vi "get_mcs_data.vi"(10 "MCS Parameters":T1={"Scan Length (Bins)"=64.0, "Dwell Time (s)"=1e-07, "Gate Channel Settings"={"Threshold (V)"=0.0, "Edge"=enum."Falling", "Input Impedence"=enum."1k Ohm"}, "Trig Channel Settings"={"Threshold (V)"=0.0, "Edge"=enum."Falling", "Input Impedence"=enum."1k Ohm"}, "Input 1 Settings"={"Threshold (V)"=0.0, "Edge"=enum."Falling", "Input Impedence"=enum."1k Ohm"}, "Input 2 Settings"={"Threshold (V)"=0.0, "Edge"=enum."Falling", "Input Impedence"=enum."1k Ohm"}, "Number of Sweeps"=0, "Number of Sequential Cycles"=0.0, "Number of Sequences"=0.0, "Sweep Preset"=FALSE, "Sequential Mode"=FALSE, "DAC 1 Ramp Settings"={"Ramp Mode"=enum."Fixed", "Ramp Start Value (V)"=0.0, "Ramp Length (Steps)"=1, "Step Width (bins)"=0, "Step Size (V)"=0.0}, "DAC 2 Output (V)"=0.0, "SYNC Output"=enum."40 MHz Clock", "ROI Min"=0, "ROI Max"=1, "Dual MCS Mode"=FALSE, "DAC 2 Toggle"=FALSE, "MCS on/off"=FALSE, "ROI Max 2"=1, "ROI Min 2"=0, "Sum ROI Only"=FALSE, "Use ROI For \nEach Loop"=FALSE} {"ROI Max 2" min=1; "ROI Min 2" min=0; "ROI Max" min=1; "ROI Min" min=0; "DAC 2 Output (V)" min=-10.0 max=10.0 step=0.00488; "DAC 1 Ramp Settings"."Step Size (V)" min=0.0 max=10.0 step=0.00244 format="%#_4g"; "DAC 1 Ramp Settings"."Step Width (bins)" min=1; "DAC 1 Ramp Settings"."Ramp Length (Steps)" min=1; "DAC 1 Ramp Settings"."Ramp Start Value (V)" min=0.0 max=10.0 step=0.00244; "Number of Sweeps" min=0 format="%.0p"; "Input 2 Settings"."Threshold (V)" min=-2.5 max=2.5 step=0.001; "Input 1 Settings"."Threshold (V)" min=-2.5 max=2.5 step=0.001; "Trig Channel Settings"."Threshold (V)" min=-2.5 max=2.5 step=0.001; "Gate Channel Settings"."Threshold (V)" min=-2.5 max=2.5 step=0.001; "Dwell Time (s)" min=1e-07 step=2.5e-08 format="%#_6p"; "Scan Length (Bins)" min=64.0 max=524288.0 format="%#_7f"}) -> (2 "2d Data":u32[][](array[numeric]))   [LabVIEW 2013]
uses:
  Controls/MCS/mcs_control_panel.ctl
  2015.07.19_Rydberg_ExpControl/Controls/MCS/mcs_channel.ctl
  Controls/MCS/ramp_control.ctl
panel:
  out "Data":u32[](array[numeric])
  out "MCA3Stst Return code":i32
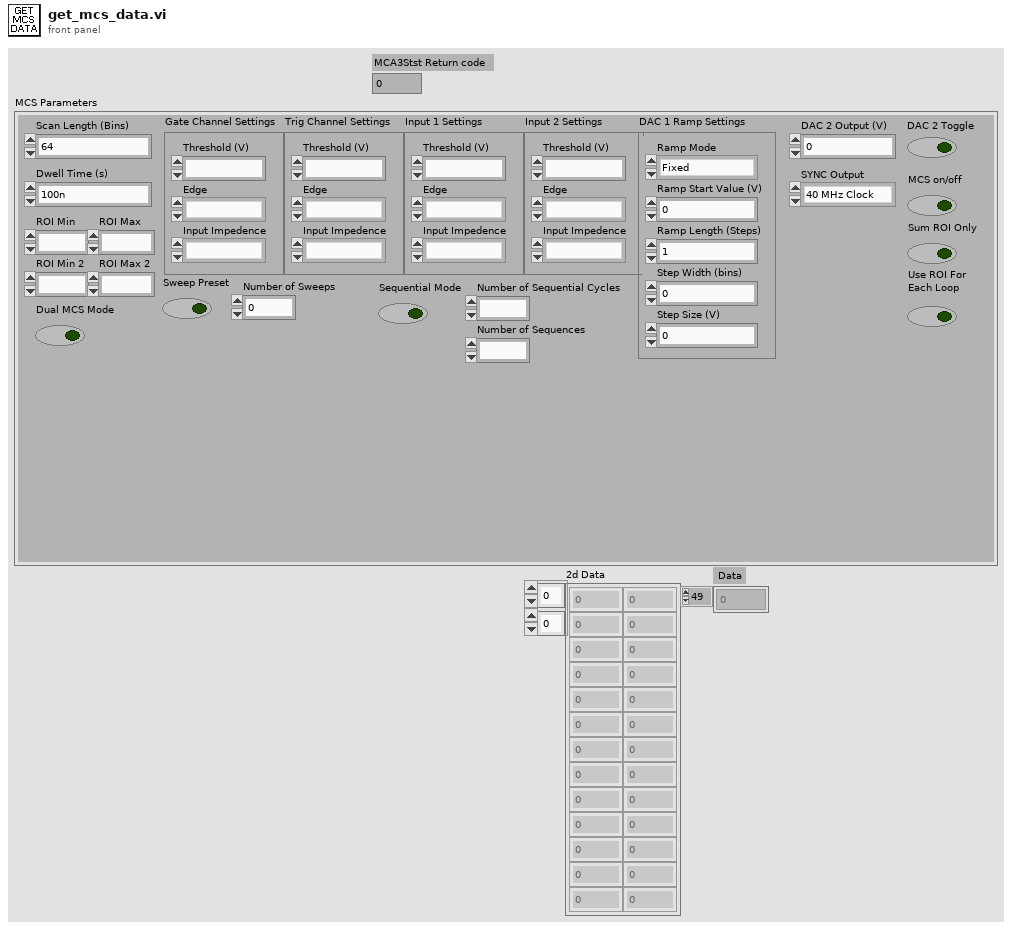
[diagram p1: front panel]
types:
  T1 = typedef "mcs_control_panel.ctl" = cluster{"Scan Length (Bins)":dbl, "Dwell Time (s)":dbl, "Gate Channel Settings":T2, "Trig Channel Settings":T2, "Input 1 Settings":T2, "Input 2 Settings":T2, "Number of Sweeps":i32, "Number of Sequential Cycles":dbl, "Number of Sequences":dbl, "Sweep Preset":bool, "Sequential Mode":bool, "DAC 1 Ramp Settings":T3, "DAC 2 Output (V)":dbl, "SYNC Output":enum16{"40 MHz Clock", "Gate Disc Signal", "Trigger Disc Signal", "Counter 1 Disc Signal", "Counter 2 Disc Signal", "Definitely Not Used", "Not Used", "1 kHz Signal", "Also Not Used", "MCS On/Off", "End of Time Bin", "Ramp Increment Trig", "Step Count Trigger", "'GO'-Line", "Ramp Down Trigger", "Logic 1"}, "ROI Min":i32, "ROI Max":i32, "Dual MCS Mode":bool, "DAC 2 Toggle":bool, "MCS on/off":bool, "ROI Max 2":i32, "ROI Min 2":i32, "Sum ROI Only":bool, "Use ROI For \nEach Loop":bool}
  T2 = typedef "mcs_channel.ctl" = cluster{"Threshold (V)":dbl, "Edge":enum16{"Falling", "Rising"}, "Input Impedence":enum16{"1k Ohm", "50 Ohm"}}
  T3 = typedef "ramp_control.ctl" = cluster{"Ramp Mode":enum16{"Fixed", "Triangle", "Sawtooth"}, "Ramp Start Value (V)":dbl, "Ramp Length (Steps)":i32, "Step Width (bins)":i32, "Step Size (V)":dbl}
  T4 = cluster{"Running":i32, "Dummy1":i32, "Realtime":dbl, "TotalSum":dbl, "RoiSum":dbl, "TotalRate":dbl, "NetSum":dbl, "Livetime(Sweeps)":dbl, "Deadtime":dbl, "Maxval":u32, "Dummy2":i32}
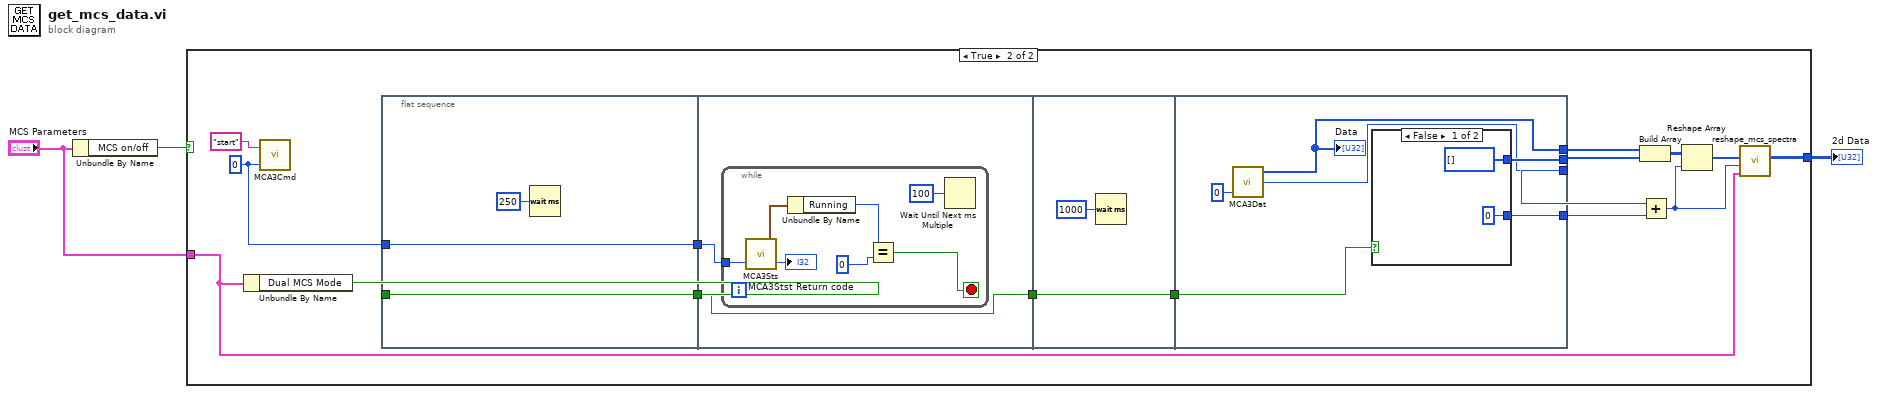
[diagram p0: block diagram]
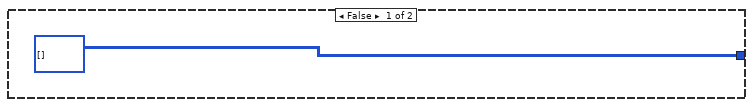
[diagram p2: hidden frame]
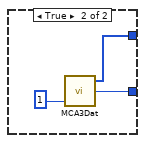
[diagram p3: hidden frame]
diagram:
  n1 = Unbundle By Name("MCS Parameters") -> ("MCS on/off"=w3:bool)
  n2 = case shown="True" w3 {
    tunnel: [u32[][] [] ("2d Data") w19] -> w1
    tunnel: "MCS Parameters" -> [_ w11]
    frame False {
    }
    frame True {
      w8 = 0 ("MCA #")
      n3 = Unbundle By Name(w11) -> ("Dual MCS Mode"=w10:bool)
      n4 = call <userlib>:"MCA3Cmd.vi"("MCA #"=w8, "Command"="start") -> ()  [unwired: 1 in, 1 out]
      n5 = flat-sequence {
        tunnel: w10 -> [w23]
        tunnel: [w23] -> w9
        tunnel: w8 -> [w22]
        tunnel: [w22] -> w7
        tunnel: [w25] -> w6
        tunnel: w9 -> [w25]
        tunnel: w7 -> [w24]
        tunnel: w6 -> [w34]
        tunnel: [w34] -> w5
        tunnel: [w36] -> w15
        tunnel: [w40] -> w14
        tunnel: [w39] -> w13
        tunnel: [w35] -> w12
        tunnel: w5 -> [w38]
        frame #0 {
          n6 = Wait (ms)(milliseconds to wait=u32 250) -> ()  [unwired: 1 out]
        }
        frame #1 {
          n7 = while {
            tunnel: w24 -> [w28]
            stop <- w27 stop-if-true
            n8 = call <userlib>:"MCA3Sts.vi"("MCD #"=w28) -> ("MCA3Stst Return code"=→"MCA3Stst Return code":i32, "MCA-3 Status"=w31:T4)  [unwired: 1 in]
            n9 = Unbundle By Name(w31) -> ("Running"=w30:i32)
            n10 = Equal?(x=w30, y=0) -> (x = y?=w27:bool)
            n11 = Wait Until Next ms Multiple(millisecond multiple=u32 100) -> ()  [unwired: 1 out]
          }
        }
        frame #2 {
          n12 = Wait (ms)(milliseconds to wait=u32 1000) -> ()  [unwired: 1 out]
        }
        frame #3 {
          n13 = call <userlib>:"MCA3Dat.vi"("MCD #"=0) -> ("Spectrum Length"=w36:i32, "Data"=w35:u32[])  [unwired: 2 in, 1 out]
          "Data" <- w35
          n14 = case shown="False" w38 {
            tunnel: [0 ("Spectrum Length") w44] -> w40
            tunnel: [u32[] [] ("Data") w43] -> w39
            frame False {
            }
            frame True {
              n15 = call <userlib>:"MCA3Dat.vi"("MCD #"=1) -> ("Spectrum Length"=w44:i32, "Data"=w43:u32[])  [unwired: 2 in, 1 out]
            }
          }
        }
      }
      n16 = Build Array(w12, w13) -> (w18:u32[][])
      n17 = Add(x=w15, y=w14) -> (x+y=w17:i32)
      n18 = Reshape Array(w18, w17) -> (w16:u32[])
      n19 = call "reshape_mcs_spectra.vi"("MCS Parameters"=w11, "Spectrum Length"=w17, "Data"=w16) -> ("2d Data"=w19:u32[][])  [unwired: 8 in]
    }
  }
  "2d Data" <- w1
